vi "project.vi"() -> ()   [LabVIEW 2020]
uses:
  <vilib>/Instr/_visa.llb/VISA Configure Serial Port (Instr).vi
panel:
  out "array":string[](array[string])
  in  "Array":string[](array[string])
  out "error out 3":errorcluster
  in  "error in":errorcluster
  in  "stop 2":bool
  in  "Ring":u16(ring) items=["Heat Index"=8, "Humidity"=7, "Temperature"=6, "MQ135 "=4, "MQ9"=2, "MQ2 "=0]
  out "Waveform Chart 2":dbl[](graph)
  out "MQ2 %               Alert               MQ9 %                Alert             MQ135 %             Alert                  Temp            Humidity %       Heat Index":dbl[][](array[numeric])
  out "read buffer":string
  in  "operation (0:open)":T1(ring)
  in  "file path (use dialog)":path
  in  "data bits (8)":u16=8 min=5 max=8 step=1
  in  "byte count":u32
  out "error out 2":errorcluster
  in  "stop":bool
  out "error out":errorcluster
  in  "access (0:read/write)":enum16{"read/write", "read-only", "write-only"}(ring)
  in  "error in (no error)":errorcluster
  in  "Port":refnum<visa-resource-name>
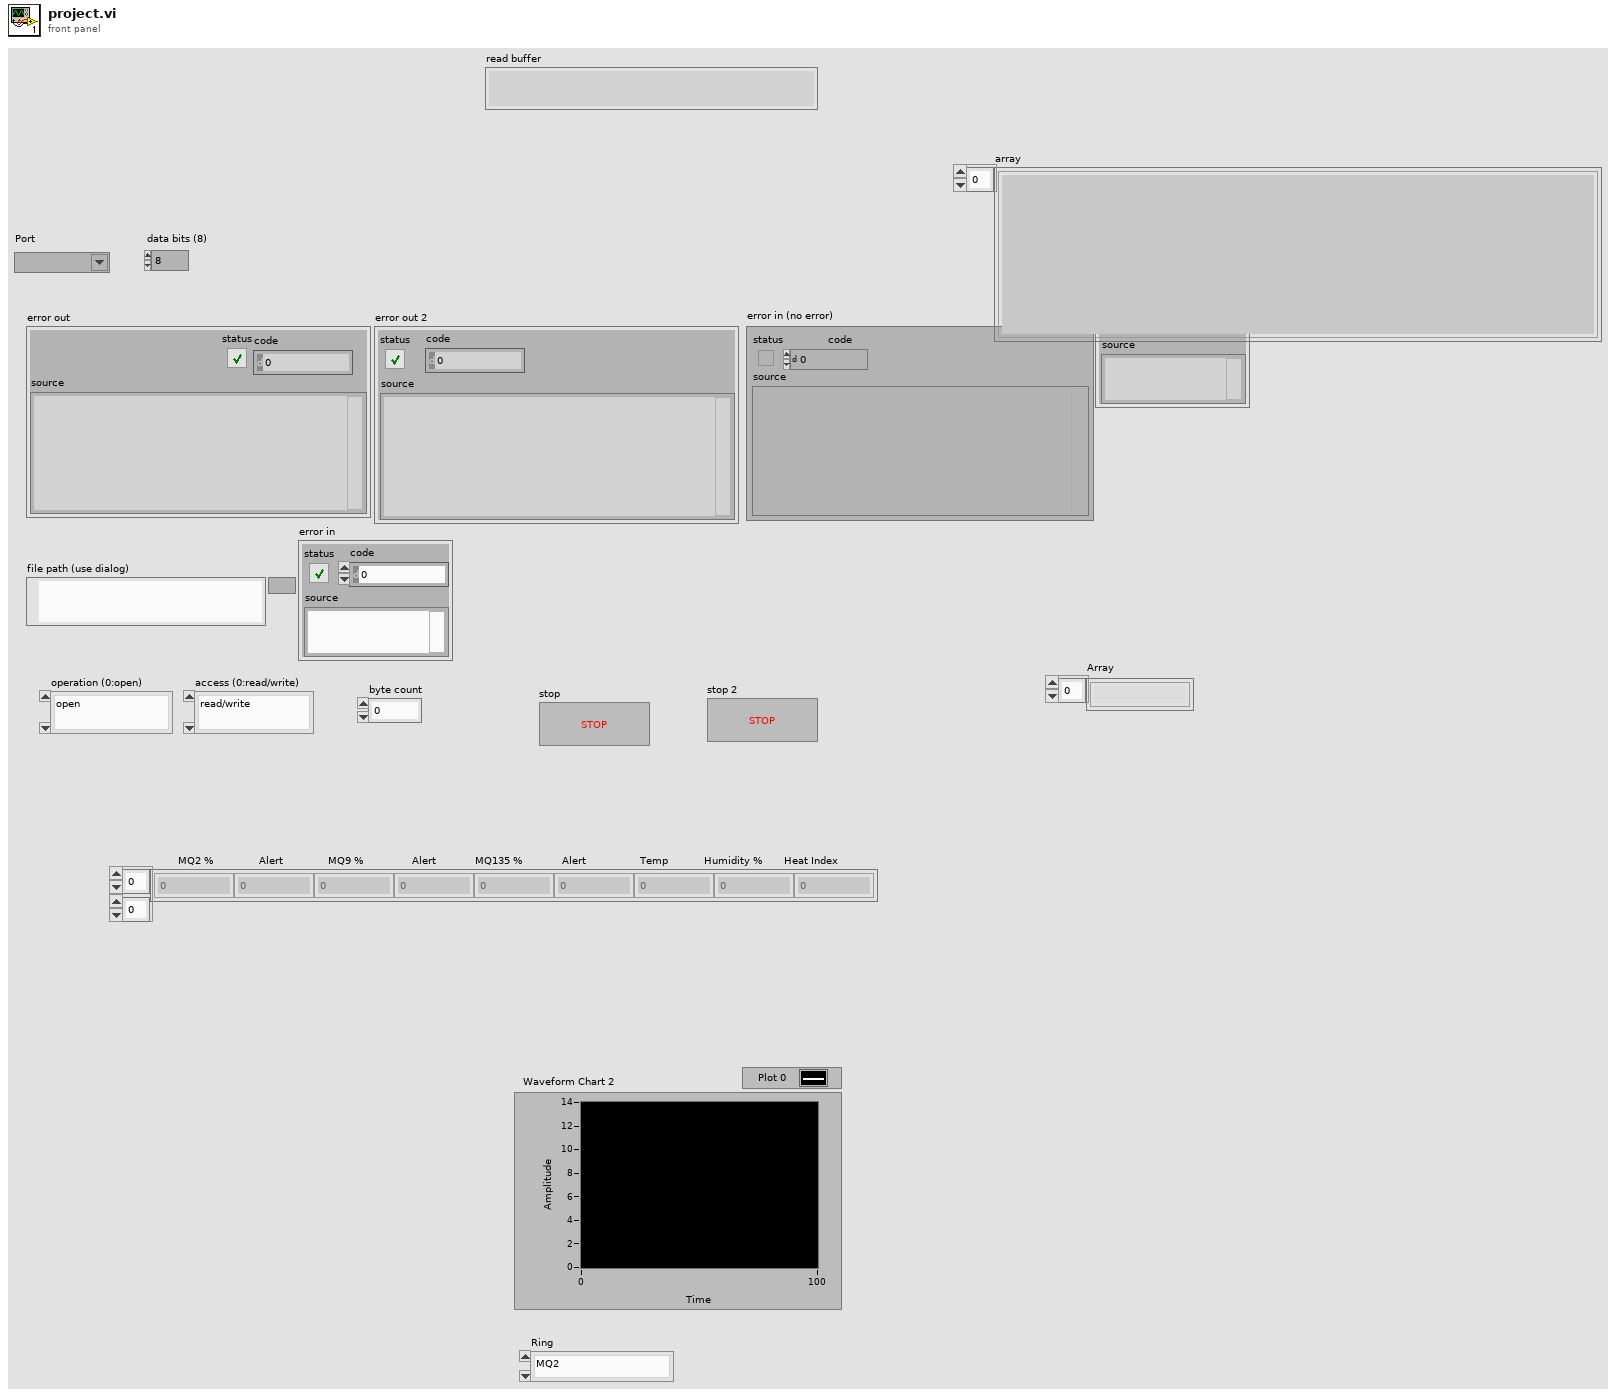
[diagram p1: front panel]
types:
  T1 = enum16{"open", "replace", "create", "open or create", "replace or create", "replace or create with confirmation"}
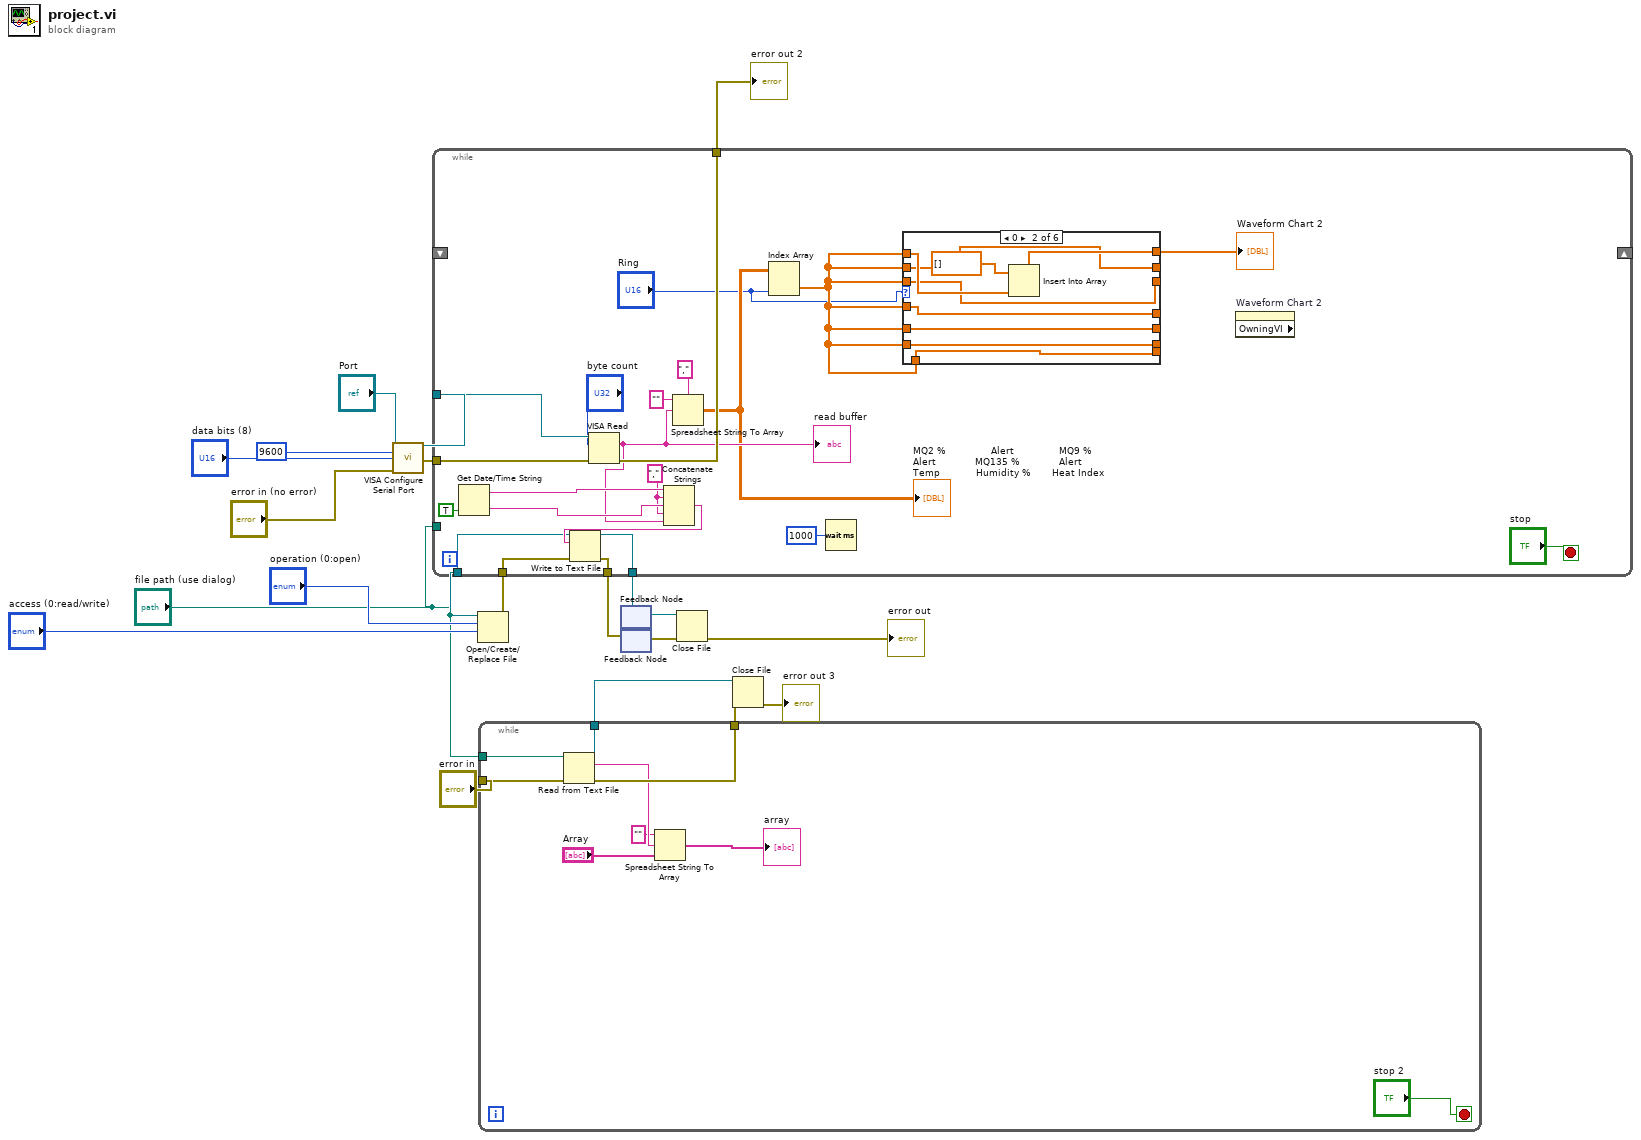
[diagram p0: block diagram]
diagram:
  n1 = call-poly "VISA Configure Serial Port"("VISA resource name"="Port", "baud rate (9600)"=u32 9600, "data bits (8)"="data bits (8)", "error in (no error)"="error in (no error)") -> ("VISA resource name out"=w18:refnum<visa-resource-name>, "error out"=w17:errorcluster)  [unwired: 10 in]
  n2 = Open/Create/Replace File(file path (use dialog)="file path (use dialog)", operation (0:open)="operation (0:open)", access (0:read/write)="access (0:read/write)") -> (refnum out=w8:refnum<file>, error out=w9:errorcluster)  [unwired: 3 in, 1 out]
  n3 = while {
    tunnel: w18 -> [w43]
    tunnel: w17 -> [w42]
    tunnel: [w38] -> w10
    tunnel: w9 -> [w35]
    tunnel: w8 -> [w26]
    tunnel: [w34] -> w7
    tunnel: [w33] -> w6
    tunnel: "file path (use dialog)" -> [_]
    shift-right: _ -> [_]
    shift-left: _ -> [_]
    stop <- "stop" stop-if-true
    w27 = "," ("string")
    n4 = Get Date/Time String(want seconds? (F)=TRUE) -> (date string=w32:string, time string=w31:string)  [unwired: 2 in]
    n5 = VISA Read(VISA resource name=w43, byte count="byte count", error in (no error)=w42) -> (read buffer=w30:string, error out=w38:errorcluster)  [unwired: 2 out]
    "read buffer" <- w30
    n6 = Concatenate Strings(w32, w27, w31, w27, w30) -> (w29:string)
    n7 = Write to Text File(file (use dialog)=w26, text=w29, error in=w35) -> (refnum out=w33:refnum<file>, error out=w34:errorcluster)  [unwired: 1 in, 1 out]
    n8 = Spreadsheet String To Array(delimiter (Tab)=",", format string="", spreadsheet string=w30) -> (array=w25:dbl[][])  [unwired: 1 in]
    "MQ2 %               Alert               MQ9 %                Alert             MQ135 %             Alert                  Temp            Humidity %       Heat Index" <- w25
    n9 = Index Array(array=w25, index (col)="Ring") -> (element=w24:dbl[])  [unwired: 1 in]
    n10 = Wait (ms)(milliseconds to wait=u32 1000) -> ()  [unwired: 1 out]
    n11 = case shown="0" "Ring" {
      tunnel: w24 -> [_ w51 _ _ _ _]
      tunnel: w24 -> [_ w49 _ _ _ _]
      tunnel: w24 -> [_ w48 _ _ _ _]
      tunnel: w24 -> [_ w47 _ _ _ _]
      tunnel: w24 -> [_ w46 _ _ _ _]
      tunnel: w24 -> [_ w45 _ _ _ _]
      tunnel: w24 -> [_ w44 _ _ _ _]
      tunnel: [_ w50 _ _ _ _] -> w22
      tunnel: [_ w49 _ _ _ _] -> _
      tunnel: [_ w48 _ _ _ _] -> _
      tunnel: [_ w47 _ _ _ _] -> _
      tunnel: [_ w46 _ _ _ _] -> _
      tunnel: [_ w45 _ _ _ _] -> _
      tunnel: [_ w44 _ _ _ _] -> _
      frame 8 {
      }
      frame 0 {
        n12 = Insert Into Array(array=dbl[] [], new element=w51) -> (w50:dbl[])  [unwired: 1 in]
      }
      frame 2 {
      }
      frame 4 {
      }
      frame 6 {
      }
      frame 7 {
      }
    }
    "Waveform Chart 2" <- w22
    n13 = property on="Waveform Chart 2" class="WFChart (strict)" props=["OwningVI"]() -> ()  [unwired: 2 in, 3 out]
  }
  "error out 2" <- w10
  n14 = while {
    tunnel: "file path (use dialog)" -> [w60]
    tunnel: "error in" -> [w59]
    tunnel: [w57] -> w4
    tunnel: [w58] -> w3
    stop <- "stop 2" stop-if-true
    n15 = Read from Text File(file (use dialog)=w60, error in=w59) -> (refnum out=w58:refnum<file>, text=w56:string, error out=w57:errorcluster)  [unwired: 2 in, 1 out]
    n16 = Spreadsheet String To Array(format string="", spreadsheet string=w56, array type (2D Dbl)="Array") -> (array=→"array":string[])  [unwired: 1 in]
  }
  n17 = feedback-in #1(w6) -> ()
  n18 = feedback #1() -> (w14:refnum<file>)  [unwired: 1 in]
  n19 = feedback-in #2(w7) -> ()
  n20 = feedback #2() -> (w13:errorcluster)  [unwired: 1 in]
  n21 = Close File(refnum=w14, error in=w13) -> (error out=→"error out":errorcluster)  [unwired: 1 out]
  n22 = Close File(refnum=w3, error in=w4) -> (error out=→"error out 3":errorcluster)  [unwired: 1 out]
